vi "End.vi"   [LabVIEW 2018, in "Toolkit.lvlib" / "Reader.lvclass"]
doc: "Finishes decoding MessagePack data. This must be called after reading all of the data to free resources and allow reuse of the object."
uses:
  Reader.lvclass
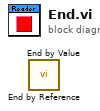
[diagram p0: block diagram]
diagram:
  n1 = call "End by Reference.vi"() -> ()  [unwired: 10 in, 2 out]
  n2 = call "End by Value.vi"() -> ()  [unwired: 10 in, 2 out]
